vi "Live window-Prevent intensity inversion.vi"(7 "Which image display?":T1, 8 "error in (no error)":errorcluster, 9 "Old value":cluster{i16, i16}(slide)={0, 2048} scale=0.0..4095.0, 11 "New value":cluster{i16, i16}(slide)={0, 2048} scale=0.0..4095.0) -> (0 "error out":errorcluster, 2 "Output setting":cluster{i16, i16}(slide)={0, 2048} scale=0.0..4095.0)   [LabVIEW 2013]
uses:
  Typedefs/Left-Right enum.ctl
  Globals/gl_Windows Ctrl refs.vi
panel:
  in  "Minimum spacing between sliders":i16=150
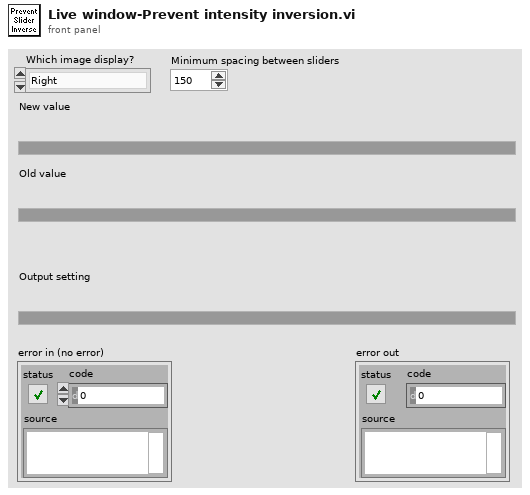
[diagram p1: front panel]
types:
  T1 = typedef "Left-Right enum.ctl" = enum16{"Right", "Left"}
  T2 = typedef "Live window-ctrl refs.ctl" = cluster{"This VI":refnum<vi>, "Pane":refnum<vi>, "Snapshot":refnum<vi>, "Left Image Palette":refnum<vi>, "Right Image Palette":refnum<vi>, "Left Channel":refnum<vi>, "Right Channel":refnum<vi>, "Left image intensity":refnum<vi>, "Right image intensity":refnum<vi>, "Left Image Display":T3, "Right Image Display":T3, "Refresh rate ind (Hz)":refnum<vi>, "Acq rate ind (Hz)":refnum<vi>, "Stop (ind)":refnum<vi>}
  T3 = typedef "Image display ref.ctl" = refnum<vi>
  T4 = cluster{"Scale.Maximum":dbl, "Scale.Minimum":dbl}
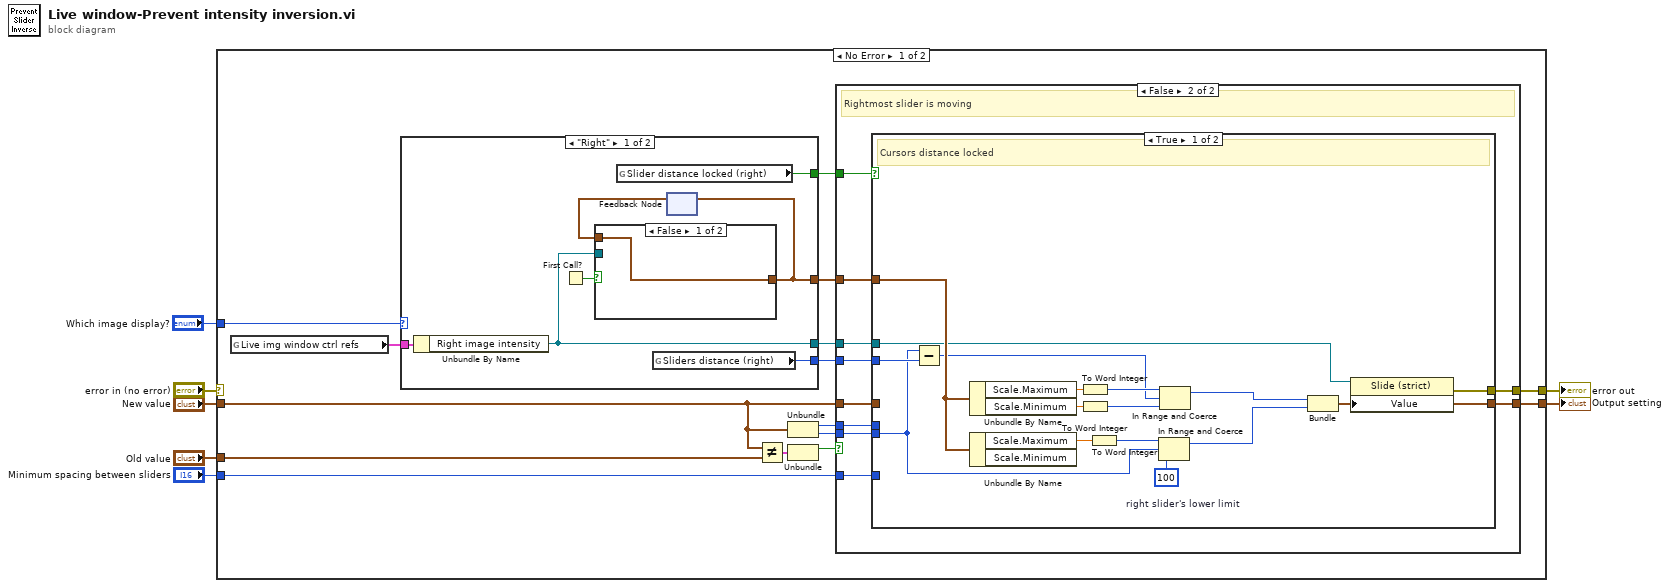
[diagram p0: block diagram]
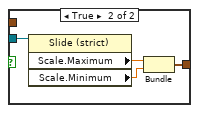
[diagram p2: hidden frame]
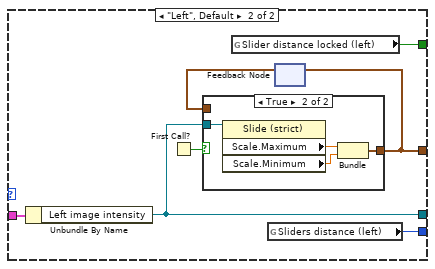
[diagram p3: hidden frame]
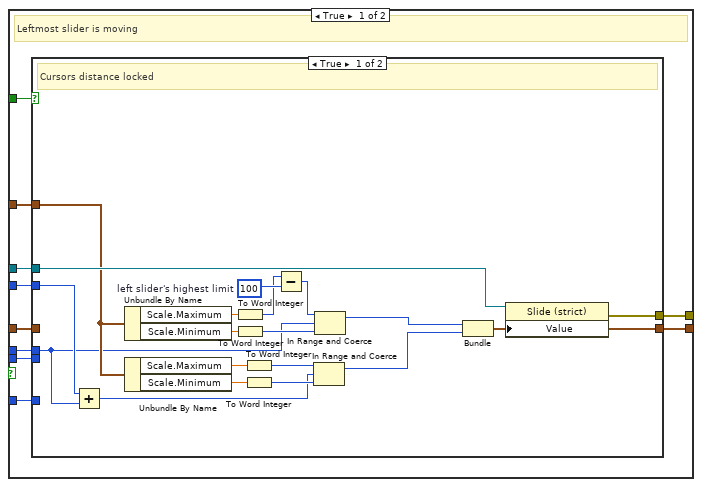
[diagram p5: hidden frame]
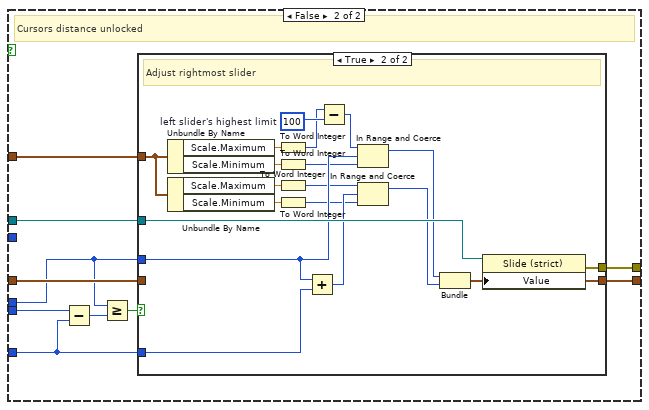
[diagram p6: hidden frame]
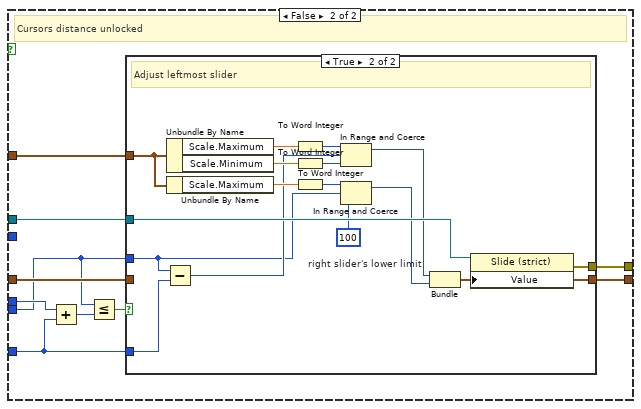
[diagram p8: hidden frame]
diagram:
  n1 = case shown="No Error" "error in (no error)" {
    selector: "error in (no error)" -> [_ w160]
    tunnel: [w14 w160] -> w6
    tunnel: "New value" -> [w20 w159]
    tunnel: "Old value" -> [w21 _]
    tunnel: [w16 w159] -> w3
    tunnel: "Which image display?" -> [w18 _]
    tunnel: "Minimum spacing between sliders" -> [w11 _]
    frame No Error {
      n2 = global read "gl_Windows Ctrl refs.vi" "Live img window ctrl refs"() -> (w19:T2)
      n3 = case shown="\"Right\"" w18 {
        tunnel: w19 -> [w29 w41]
        tunnel: [w26 w40] -> w15
        tunnel: [w25 w37] -> w10
        tunnel: [w24 w36] -> w9
        tunnel: [w23 w35] -> w8
        frame "Right" {
          n4 = Unbundle By Name(w29) -> ("Right image intensity"=w26:refnum<vi>)
          n5 = First Call?() -> (First Call?: T/F=w27:bool)
          n6 = global read "gl_Windows Ctrl refs.vi" "Slider distance locked (right)"() -> (w24:bool)
          n7 = global read "gl_Windows Ctrl refs.vi" "Sliders distance (right)"() -> (w23:i16)
          n8 = feedback #1() -> (w28:T4)  [unwired: 1 in]
          n9 = case shown="False" w27 {
            tunnel: w26 -> [_ w34]
            tunnel: [w30 w31] -> w25
            tunnel: w28 -> [w30 _]
            frame False {
            }
            frame True {
              n10 = property class="Slide (strict)"(reference=w34) -> ("Scale.Maximum"=w33:dbl, "Scale.Minimum"=w32:dbl)  [unwired: 1 in, 2 out]
              n11 = Bundle("Scale.Maximum"=w33, "Scale.Minimum"=w32) -> (w31:T4)  [unwired: 1 in]
            }
          }
          n12 = feedback-in #1(w25) -> ()
        }
        frame "Left", Default {
          n13 = Unbundle By Name(w41) -> ("Left image intensity"=w40:refnum<vi>)
          n14 = First Call?() -> (First Call?: T/F=w38:bool)
          n15 = global read "gl_Windows Ctrl refs.vi" "Slider distance locked (left)"() -> (w36:bool)
          n16 = global read "gl_Windows Ctrl refs.vi" "Sliders distance (left)"() -> (w35:i16)
          n17 = feedback #2() -> (w39:T4)  [unwired: 1 in]
          n18 = case shown="True" w38 {
            tunnel: w40 -> [_ w46]
            tunnel: [w42 w43] -> w37
            tunnel: w39 -> [w42 _]
            frame False {
            }
            frame True {
              n19 = property class="Slide (strict)"(reference=w46) -> ("Scale.Maximum"=w45:dbl, "Scale.Minimum"=w44:dbl)  [unwired: 1 in, 2 out]
              n20 = Bundle("Scale.Maximum"=w45, "Scale.Minimum"=w44) -> (w43:T4)  [unwired: 1 in]
            }
          }
          n21 = feedback-in #2(w37) -> ()
        }
      }
      n22 = Not Equal?(x=w20, y=w21) -> (x != y?=w22:cluster{bool, bool})
      n23 = Unbundle(w20) -> (w13:i16, w12:i16)
      n24 = Unbundle(w22) -> (w17:bool)  [unwired: 1 out]
      n25 = case shown="False" w17 {
        tunnel: w12 -> [w56 w109]
        tunnel: w13 -> [w50 w110]
        tunnel: w11 -> [w55 w115]
        tunnel: [w54 w114] -> w16
        tunnel: w20 -> [w53 w113]
        tunnel: w15 -> [w52 w112]
        tunnel: [w51 w111] -> w14
        tunnel: w10 -> [w49 w108]
        tunnel: w9 -> [w48 w107]
        tunnel: w8 -> [w47 w106]
        frame True {
          # "Leftmost slider is moving"
          n26 = case shown="True" w48 {
            tunnel: w56 -> [_ w83]
            tunnel: w55 -> [_ w82]
            tunnel: [w75 w81] -> w54
            tunnel: w53 -> [_ w80]
            tunnel: w52 -> [w74 w79]
            tunnel: [w73 w78] -> w51
            tunnel: w50 -> [w58 w77]
            tunnel: w49 -> [w59 w76]
            tunnel: w47 -> [w72 _]
            frame True {
              w64 = i16 100  # left slider's highest limit
              # "Cursors distance locked"
              n27 = Add(x=w72, y=w58) -> (x+y=w66:i16)
              n28 = Unbundle By Name(w59) -> ("Scale.Maximum"=w62:dbl, "Scale.Minimum"=w65:dbl)
              n29 = Unbundle By Name(w59) -> ("Scale.Maximum"=w71:dbl, "Scale.Minimum"=w70:dbl)
              n30 = To Word Integer(number=w62) -> (16bit integer=w61:i16)
              n31 = To Word Integer(number=w65) -> (16bit integer=w60:i16)
              n32 = To Word Integer(number=w71) -> (16bit integer=w67:i16)
              n33 = To Word Integer(number=w70) -> (16bit integer=w69:i16)
              n34 = Subtract(x=w61, y=w64) -> (x-y=w63:i16)
              n35 = In Range and Coerce(upper limit=w67, x=w66, lower limit=w69) -> (coerced(x)=w68:i16)  [unwired: 1 out]
              n36 = In Range and Coerce(upper limit=w63, x=w58, lower limit=w60) -> (coerced(x)=w57:i16)  [unwired: 1 out]
              n37 = Bundle(w57, w68) -> (w75:cluster{i16, i16})  [unwired: 1 in]
              n38 = property class="Slide (strict)"(reference=w74, "Value"=w75) -> (error out=w73:errorcluster)  [unwired: 1 in, 1 out]
            }
            frame False {
              # "Cursors distance unlocked"
              n39 = Subtract(x=w83, y=w82) -> (x-y=w85:i16)
              n40 = Greater Or Equal?(x=w77, y=w85) -> (x >= y?=w84:bool)
              n41 = case shown="True" w84 {
                tunnel: w77 -> [_ w94]
                tunnel: w82 -> [_ w105]
                tunnel: [w86 w104] -> w81
                tunnel: w80 -> [w86 _]
                tunnel: w79 -> [_ w103]
                tunnel: [_ w102] -> w78
                tunnel: w76 -> [_ w99]
                frame False {
                  # "Idle"
                }
                frame True {
                  w97 = i16 100  # left slider's highest limit
                  # "Adjust rightmost slider"
                  n42 = Unbundle By Name(w99) -> ("Scale.Maximum"=w95:dbl, "Scale.Minimum"=w101:dbl)
                  n43 = Unbundle By Name(w99) -> ("Scale.Maximum"=w98:dbl, "Scale.Minimum"=w100:dbl)
                  n44 = To Word Integer(number=w95) -> (16bit integer=w90:i16)
                  n45 = To Word Integer(number=w101) -> (16bit integer=w89:i16)
                  n46 = To Word Integer(number=w98) -> (16bit integer=w88:i16)
                  n47 = To Word Integer(number=w100) -> (16bit integer=w87:i16)
                  n48 = Add(x=w94, y=w105) -> (x+y=w93:i16)
                  n49 = Subtract(x=w90, y=w97) -> (x-y=w96:i16)
                  n50 = In Range and Coerce(upper limit=w96, x=w94, lower limit=w89) -> (coerced(x)=w91:i16)  [unwired: 1 out]
                  n51 = In Range and Coerce(upper limit=w88, x=w93, lower limit=w87) -> (coerced(x)=w92:i16)  [unwired: 1 out]
                  n52 = Bundle(w91, w92) -> (w104:cluster{i16, i16})  [unwired: 1 in]
                  n53 = property class="Slide (strict)"(reference=w103, "Value"=w104) -> (error out=w102:errorcluster)  [unwired: 1 in, 1 out]
                }
              }
            }
          }
        }
        frame False {
          # "Rightmost slider is moving"
          n54 = case shown="True" w107 {
            tunnel: w115 -> [_ w139]
            tunnel: [w117 w138] -> w114
            tunnel: w113 -> [_ w137]
            tunnel: w112 -> [w123 w136]
            tunnel: [w116 w135] -> w111
            tunnel: w110 -> [_ w134]
            tunnel: w109 -> [w119 w133]
            tunnel: w108 -> [w124 w132]
            tunnel: w106 -> [w120 _]
            frame True {
              w122 = i16 100  # right slider's lower limit
              # "Cursors distance locked"
              n55 = Subtract(x=w119, y=w120) -> (x-y=w118:i16)
              n56 = Unbundle By Name(w124) -> ("Scale.Maximum"=w127:dbl, "Scale.Minimum"=w128:dbl)
              n57 = Unbundle By Name(w124) -> ("Scale.Maximum"=w131:dbl)  [unwired: 1 out]
              n58 = To Word Integer(number=w127) -> (16bit integer=w121:i16)
              n59 = To Word Integer(number=w128) -> (16bit integer=w126:i16)
              n60 = To Word Integer(number=w131) -> (16bit integer=w129:i16)
              n61 = In Range and Coerce(upper limit=w129, x=w119, lower limit=w122) -> (coerced(x)=w130:i16)  [unwired: 1 out]
              n62 = In Range and Coerce(upper limit=w121, x=w118, lower limit=w126) -> (coerced(x)=w125:i16)  [unwired: 1 out]
              n63 = Bundle(w125, "right slider's lower limit"=w130) -> (w117:cluster{i16, "right slider's lower limit":i16})  [unwired: 1 in]
              n64 = property class="Slide (strict)"(reference=w123, "Value"=w117) -> (error out=w116:errorcluster)  [unwired: 1 in, 1 out]
            }
            frame False {
              # "Cursors distance unlocked"
              n65 = Add(x=w134, y=w139) -> (x+y=w141:i16)
              n66 = Less Or Equal?(x=w133, y=w141) -> (x <= y?=w140:bool)
              n67 = case shown="True" w140 {
                tunnel: w133 -> [_ w148]
                tunnel: w139 -> [_ w151]
                tunnel: [w142 w158] -> w138
                tunnel: w137 -> [w142 _]
                tunnel: w136 -> [_ w157]
                tunnel: [_ w156] -> w135
                tunnel: w132 -> [_ w152]
                frame False {
                  # "Idle"
                }
                frame True {
                  w150 = i16 100  # right slider's lower limit
                  # "Adjust leftmost slider"
                  n68 = Subtract(x=w148, y=w151) -> (x-y=w149:i16)
                  n69 = Unbundle By Name(w152) -> ("Scale.Maximum"=w155:dbl, "Scale.Minimum"=w154:dbl)
                  n70 = Unbundle By Name(w152) -> ("Scale.Maximum"=w153:dbl)
                  n71 = To Word Integer(number=w155) -> (16bit integer=w145:i16)
                  n72 = To Word Integer(number=w154) -> (16bit integer=w144:i16)
                  n73 = To Word Integer(number=w153) -> (16bit integer=w143:i16)
                  n74 = In Range and Coerce(upper limit=w145, x=w149, lower limit=w144) -> (coerced(x)=w146:i16)  [unwired: 1 out]
                  n75 = In Range and Coerce(upper limit=w143, x=w148, lower limit=w150) -> (coerced(x)=w147:i16)  [unwired: 1 out]
                  n76 = Bundle(w146, "right slider's lower limit"=w147) -> (w158:cluster{i16, "right slider's lower limit":i16})  [unwired: 1 in]
                  n77 = property class="Slide (strict)"(reference=w157, "Value"=w158) -> (error out=w156:errorcluster)  [unwired: 1 in, 1 out]
                }
              }
            }
          }
        }
      }
    }
    frame Error {
    }
  }
  "error out" <- w6
  "Output setting" <- w3
